vi "ASCII_Division.vi"(11 "字符串":string) -> (0 "蜂鸣器":string="CC", 1 "键盘锁":string="CC", 2 "On/Off":string="CC", 3 "测量模式":string="CC", 8 "过压":string="CC", 9 "过温":string="CC", 10 "CC/CV":string="CC")   [LabVIEW 2014]
panel:
  out "x << y":i32
  out "十六进制整型字符串":string
  out "*(类型 *) &x":i32
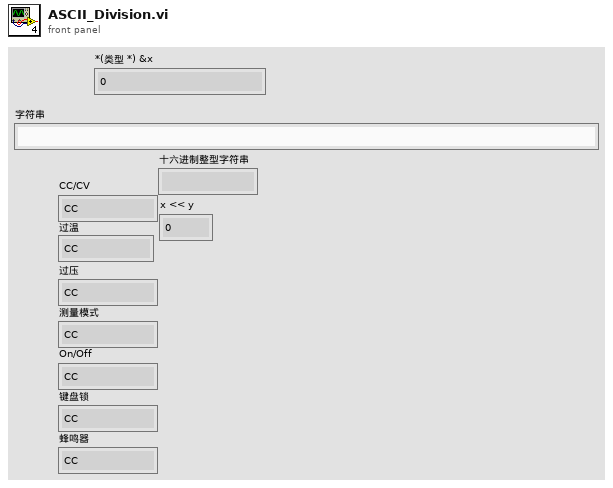
[diagram p1: front panel]
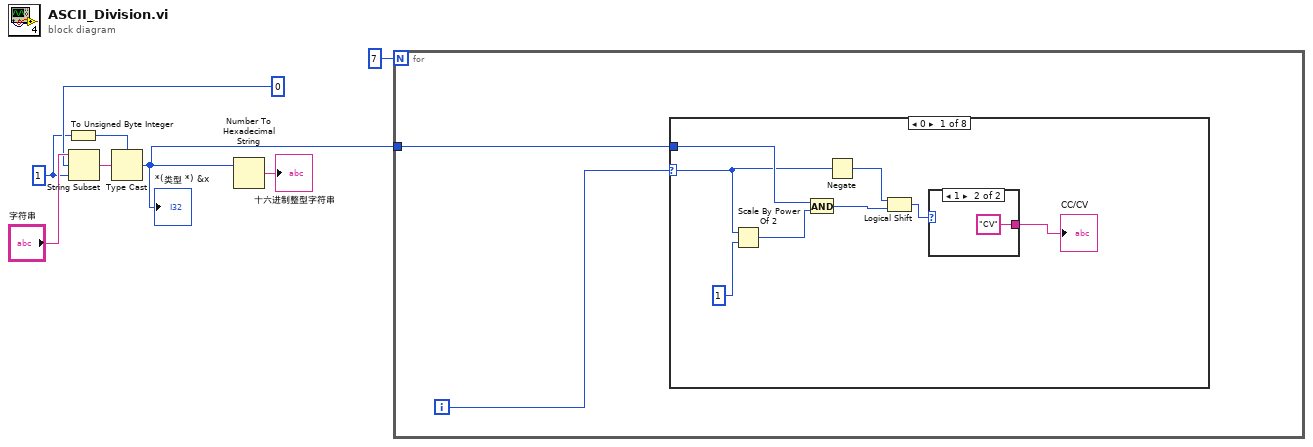
[diagram p0: block diagram]
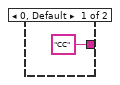
[diagram p2: hidden frame]
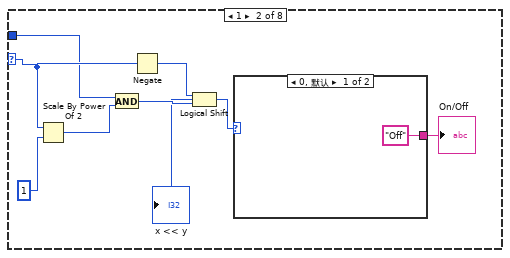
[diagram p3: hidden frame]
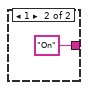
[diagram p4: hidden frame]
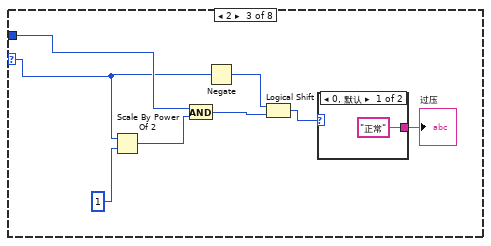
[diagram p5: hidden frame]
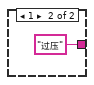
[diagram p6: hidden frame]
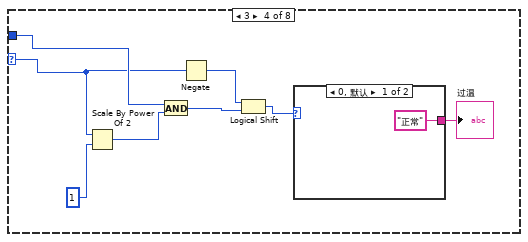
[diagram p7: hidden frame]
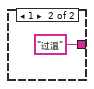
[diagram p8: hidden frame]
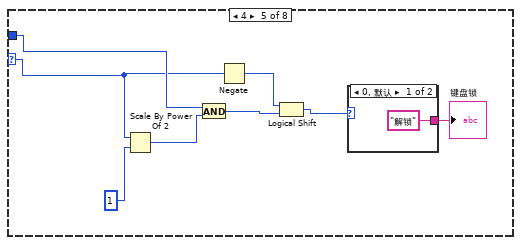
[diagram p9: hidden frame]
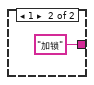
[diagram p10: hidden frame]
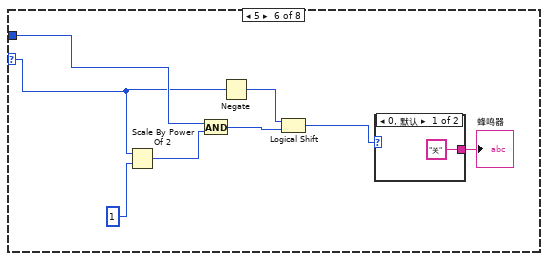
[diagram p11: hidden frame]
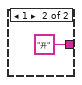
[diagram p12: hidden frame]
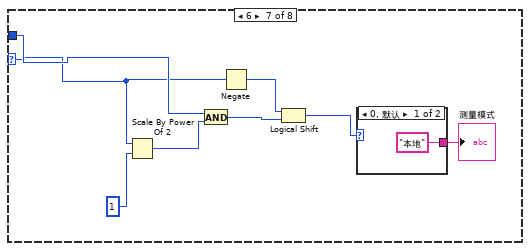
[diagram p13: hidden frame]
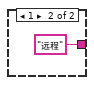
[diagram p14: hidden frame]
diagram:
  w3 = 1
  n1 = To Unsigned Byte Integer(number=w3) -> (unsigned 8bit integer=w2:u8)
  n2 = String Subset(string="字符串", offset (0)=0, length (rest)=w3) -> (substring=w5:string)
  n3 = Type Cast(type=w2, x=w5) -> (*(type *) &x=w1:u8)
  "*(类型 *) &x" <- w1
  n4 = Number To Hexadecimal String(2:w1) -> (0:→"十六进制整型字符串":string)  [unwired: 1 in]
  n5 = for {
    N: 7 -> [_]
    tunnel: w1 -> [w9]
    i -> [w10]
    n6 = case shown="0" w10 {
      selector: w10 -> [w13 w23 w31 w41 w51 w61 w71 _]
      tunnel: w9 -> [w17 w22 w32 w42 w52 w62 w72 _]
      frame 0 {
        n7 = Scale By Power Of 2(n=w13, x=1) -> (x*2^n=w16:i32)
        n8 = And(x=w17, y=w16) -> (x .and. y?=w14:i32)
        n9 = Negate(x=w13) -> (-x=w12:i32)
        n10 = Logical Shift(y=w12, x=w14) -> (x << y=w11:i32)
        n11 = case shown="1" w11 {
          tunnel: ["CC" "CV"] -> w18
          frame 0, Default {
          }
          frame 1 {
          }
        }
        "CC/CV" <- w18
      }
      frame 1 {
        n12 = Scale By Power Of 2(n=w23, x=1) -> (x*2^n=w27:i32)
        n13 = And(x=w22, y=w27) -> (x .and. y?=w25:i32)
        n14 = Negate(x=w23) -> (-x=w24:i32)
        n15 = Logical Shift(y=w24, x=w25) -> (x << y=w21:i32)
        "x << y" <- w21
        n16 = case shown="0, 默认" w21 {
          tunnel: ["Off" "On"] -> w28
          frame 0, Default {
          }
          frame 1 {
          }
        }
        "On/Off" <- w28
      }
      frame 2 {
        n17 = Scale By Power Of 2(n=w31, x=1) -> (x*2^n=w37:i32)
        n18 = And(x=w32, y=w37) -> (x .and. y?=w35:i32)
        n19 = Negate(x=w31) -> (-x=w34:i32)
        n20 = Logical Shift(y=w34, x=w35) -> (x << y=w33:i32)
        n21 = case shown="0, 默认" w33 {
          tunnel: ["正常" "过压"] -> w38
          frame 0, Default {
          }
          frame 1 {
          }
        }
        "过压" <- w38
      }
      frame 3 {
        n22 = Scale By Power Of 2(n=w41, x=1) -> (x*2^n=w47:i32)
        n23 = And(x=w42, y=w47) -> (x .and. y?=w45:i32)
        n24 = Negate(x=w41) -> (-x=w44:i32)
        n25 = Logical Shift(y=w44, x=w45) -> (x << y=w43:i32)
        n26 = case shown="0, 默认" w43 {
          tunnel: ["正常" "过温"] -> w48
          frame 0, Default {
          }
          frame 1 {
          }
        }
        "过温" <- w48
      }
      frame 4 {
        n27 = Scale By Power Of 2(n=w51, x=1) -> (x*2^n=w57:i32)
        n28 = And(x=w52, y=w57) -> (x .and. y?=w55:i32)
        n29 = Negate(x=w51) -> (-x=w54:i32)
        n30 = Logical Shift(y=w54, x=w55) -> (x << y=w53:i32)
        n31 = case shown="0, 默认" w53 {
          tunnel: ["解锁" "加锁"] -> w58
          frame 0, Default {
          }
          frame 1 {
          }
        }
        "键盘锁" <- w58
      }
      frame 5 {
        n32 = Scale By Power Of 2(n=w61, x=1) -> (x*2^n=w67:i32)
        n33 = And(x=w62, y=w67) -> (x .and. y?=w65:i32)
        n34 = Negate(x=w61) -> (-x=w64:i32)
        n35 = Logical Shift(y=w64, x=w65) -> (x << y=w63:i32)
        n36 = case shown="0, 默认" w63 {
          tunnel: ["关" "开"] -> w68
          frame 0, Default {
          }
          frame 1 {
          }
        }
        "蜂鸣器" <- w68
      }
      frame 6 {
        n37 = Scale By Power Of 2(n=w71, x=1) -> (x*2^n=w77:i32)
        n38 = And(x=w72, y=w77) -> (x .and. y?=w75:i32)
        n39 = Negate(x=w71) -> (-x=w74:i32)
        n40 = Logical Shift(y=w74, x=w75) -> (x << y=w73:i32)
        n41 = case shown="0, 默认" w73 {
          tunnel: ["本地" "远程"] -> w78
          frame 0, Default {
          }
          frame 1 {
          }
        }
        "测量模式" <- w78
      }
      frame 7, Default {
      }
    }
  }
